vi "DMCConfigurator2.vi"() -> ()   [LabVIEW 2015]
panel:
  in  "Delete":bool
  in  "Move down":bool
  in  "Move up":bool
  in  "Configuration":u16(ring) items=["Standard", ""]
  in  "DMC elements":i32(listbox)
  in  "Variables":T1(ring)
  in  "Type":enum16{"Custom Text", "Variable"}(ring)
  in  "#Digits":dbl
  in  "Custom Text":string
  in  "DMC":string
  in  "Add":bool
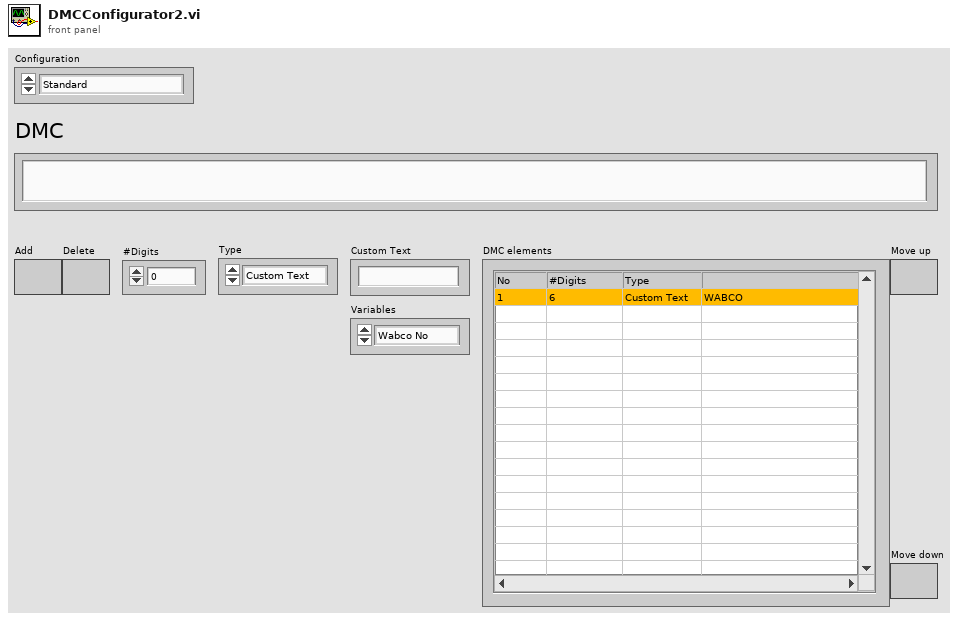
[diagram p1: front panel]
types:
  T1 = enum16{"Wabco No", "Client No", "Serial", "Date"}
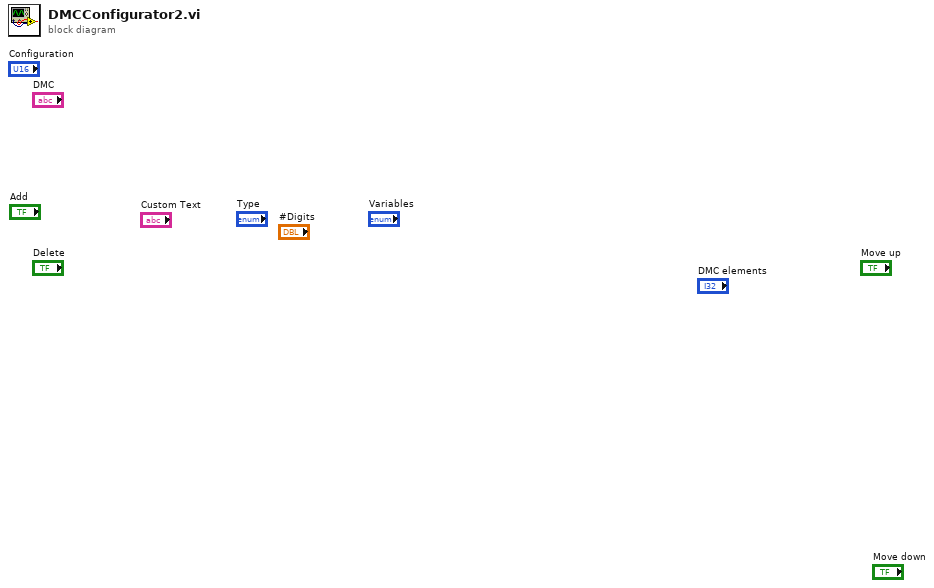
[diagram p0: block diagram]
diagram:
